vi "Get Waveform Type Enum from TD.vi"(4 "Type Descriptor":T1) -> (1 "Waveform Subtype Enum":T2 format="%.0x")   [LabVIEW 2020]
doc: "Gets a Waveform Subtype Enumeration from a Type Descriptor Array."
uses:
  Waveform Subtype Enum.ctl
  Type Descriptor.ctl
panel:
  # "Please visit http://www.OpenG.org to learn about the\nOpen Source LabVIEW software movement.\n\nNOTICE -- YOU MUST LEAVE THIS NOTICE IN PLACE.  PER THE TERMS OF THE LICENSE BELOW, YOU MAY SUBLICENSE THIS SOFTWARE \nIN ANY WAY THAT DOES NOT CONFLICT WITH THIS LICENSE.\n\n### BSD License (http://www.opensource.org/licenses/bsd-license.php) Begin ###\n \nCopyright (c) 2002-2011, Jim Kring <jim@jimkring.com>\nCopyright (c) 2011, Jonathon Green <jg@jgcode.net>\n\nAll rights reserved.\n\nRedistribution and use in source and binary forms, with or without modification, are permitted provided that the following conditions are met:\n\n    * Redistributions of source code must retain the above copyright notice, this list of conditions and the following disclaimer.\n    * Redistributions in binary form must reproduce the above copyright notice, this list of conditions and the following disclaimer in the \n       documentation and/or other materials provided with the distribution.\n    * Neither the name of SciWare, James Kring, Inc., nor the names of its contributors may be used to endorse or promote products derived \n       from this software without specific prior written permission.\n\nTHIS SOFTWARE IS PROVIDED BY THE COPYRIGHT HOLDERS AND CONTRIBUTORS \"AS IS\" AND ANY EXPRESS OR IMPLIED WARRANTIES, \nINCLUDING, BUT NOT LIMITED TO, THE IMPLIED WARRANTIES OF MERCHANTABILITY AND FITNESS FOR A PARTICULAR PURPOSE ARE \nDISCLAIMED. IN NO EVENT SHALL THE COPYRIGHT OWNER OR CONTRIBUTORS BE LIABLE FOR ANY DIRECT, INDIRECT, INCIDENTAL,\n SPECIAL, EXEMPLARY, OR CONSEQUENTIAL DAMAGES (INCLUDING, BUT NOT LIMITED TO, PROCUREMENT OF SUBSTITUTE GOODS OR \nSERVICES; LOSS OF USE, DATA, OR PROFITS; OR BUSINESS INTERRUPTION) HOWEVER CAUSED AND ON ANY THEORY OF LIABILITY, \nWHETHER IN CONTRACT, STRICT LIABILITY, OR TORT (INCLUDING NEGLIGENCE OR OTHERWISE) ARISING IN ANY WAY OUT OF THE USE \nOF THIS SOFTWARE, EVEN IF ADVISED OF THE POSSIBILITY OF SUCH DAMAGE.\n\n### BSD License End ###"
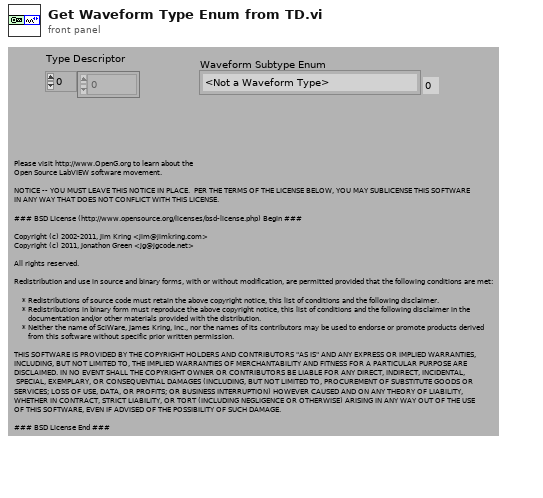
[diagram p1: front panel]
types:
  T1 = typedef "Type Descriptor.ctl" = i16[]
  T2 = typedef "Waveform Subtype Enum.ctl" = enum8{"<Not a Waveform Type>", "0x01", "Analog 16-bit signed", "Analog Double-Precision", "0x04", "Analog Single Precision", "Timestamp", "Digital Data", "Digital Waveform", "Dynamic Data", "Analog Extended-Precision", "Analog 8-bit unsigned", "Analog 16-bit unsigned", "Analog 32-bit unsigned", "Analog 8-bit signed", "Analog 32-bit signed", "Analog Complex Single-Precision", "Analog Complex Double-Precision", "Analog Complex Extended Precision", "Analog 64-bit signed", "Analog 64-bit unsigned"}
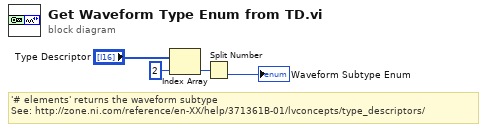
[diagram p0: block diagram]
diagram:
  # "'# elements' returns the waveform subtype\nSee: http://zone.ni.com/reference/en-XX/help/371361B-01/lvconcepts/type_descriptors/"
  n1 = Index Array(array="Type Descriptor", index=2) -> (element=w2:i16)
  n2 = Split Number(x=w2) -> (lo(x)=→"Waveform Subtype Enum":u8)  [unwired: 1 out]
